vi "LoadInstrFunc.vi"(8 "ErrorIn(No Error)":errorcluster caption="entrée d'erreur (pas d'erreur)", 9 "New Instr":bool, 10 "LoadInstr":T1, 11 "Experiment.lvclass":refnum<class "Experiment.lvclass">) -> (0 "sortie d'erreur":errorcluster, 3 "Experiment.lvclass Out":refnum<class "Experiment.lvclass">)   [LabVIEW 2019, in "Experiment.lvclass"]
uses:
  Experiment.lvclass
  LoadInstr.ctl
  Experiment.lvclass/Experiment.ctl
  DevicesClass/BaseDevice/BaseDevice.lvclass
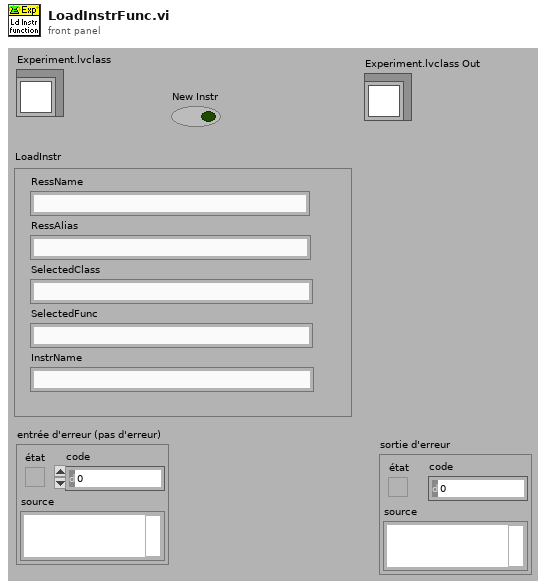
[diagram p1: front panel]
types:
  T1 = typedef "LoadInstr.ctl" = cluster{"SelectedClass":string, "SelectedFunc":string, "InstrName":string, "RessAlias":string, "RessName":string}
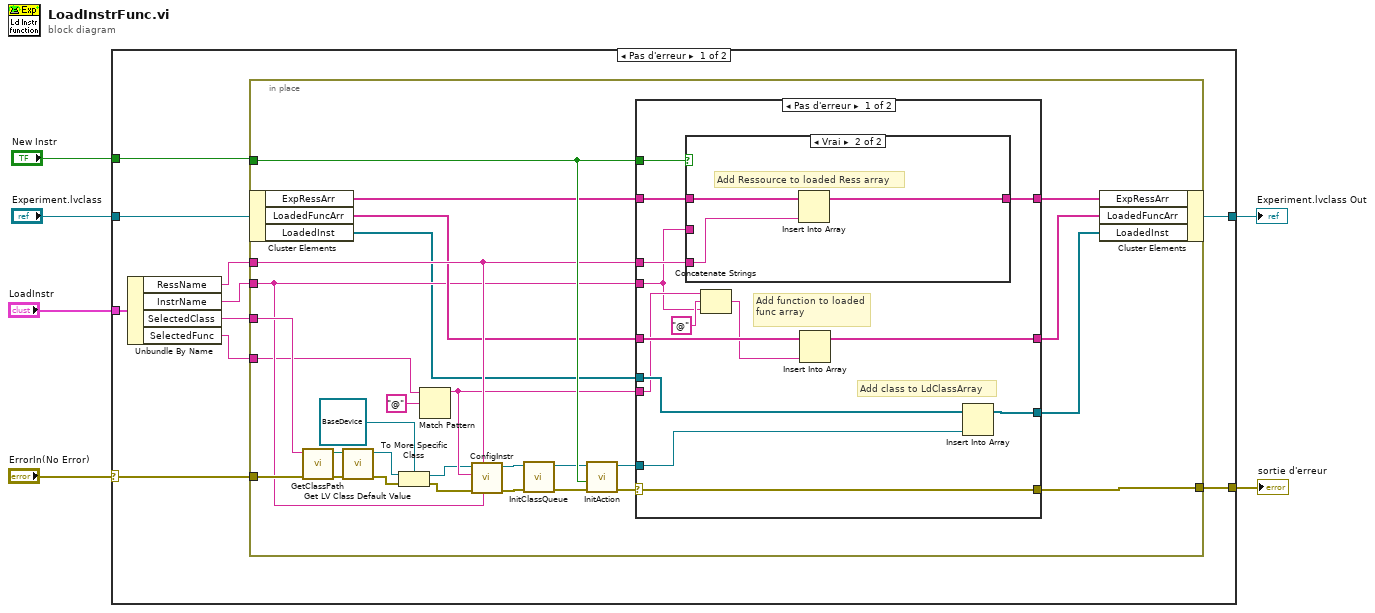
[diagram p0: block diagram]
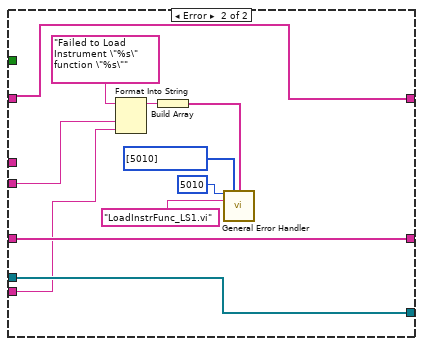
[diagram p3: hidden frame]
diagram:
  n1 = case shown="Pas d'erreur" "ErrorIn(No Error)" {
    selector: "ErrorIn(No Error)" -> [w16 w75]
    tunnel: [w15 w75] -> w5
    tunnel: "New Instr" -> [w14 _]
    tunnel: "Experiment.lvclass" -> [w12 w74]
    tunnel: [w13 w74] -> w2
    tunnel: "LoadInstr" -> [w7 _]
    frame No Error {
      n2 = Unbundle By Name(w7) -> ("RessName"=w11:string, "InstrName"=w10:string, "SelectedClass"=w9:string, "SelectedFunc"=w8:string)
      n3 = in-place {
        in-place-border: w16 -> [w40]
        in-place-border: w9 -> [w39]
        in-place-border: w11 -> [w33]
        in-place-border: w8 -> [w26]
        in-place-border: w10 -> [w28]
        in-place-border: [w38] -> w15
        in-place-border: w14 -> [w37]
        n4 = in-place-cluster #1(w12) -> ("ExpRessArr"=w34:string[], "LoadedFuncArr"=w30:string[], "LoadedInst"=w17:refnum<class "BaseDevice.lvclass">[])
        n5 = call "GetClassPath.vi"("error in (no error)"=w40, "ClassName"=w39) -> ("error out"=w41:errorcluster, "ClassPath"=w42:path)  [unwired: 7 in, 1 out]
        n6 = call <vilib>:"Get LV Class Default Value.vi"("error in (no error)"=w41, "class path"=w42) -> ("error out"=w23:errorcluster, "object"=w44:refnum<class>)  [unwired: 8 in]
        n7 = To More Specific Class(target class=refnum<class "BaseDevice.lvclass"> refnum ("Device.lvclass"), reference=w44, error in=w23) -> (specific class reference=w24:refnum<class "BaseDevice.lvclass">, error out=w22:errorcluster)
        n8 = Match Pattern(string=w26, regular expression="@" ("chaîne")) -> (before substring=w25:string)  [unwired: 1 in, 3 out]
        n9 = call-dynamic "ConfigInstr.vi"("InstrumentName"=w28, "VisaRessIn"=w33, "error in (no error)"=w22, "Function"=w25, "Device en entrée"=w24) -> ("error out"=w21:errorcluster, "Device en sortie"=w19:refnum<class "BaseDevice.lvclass">)  [unwired: 5 in]
        n10 = call "InitClassQueue.vi"("ErrorIn(No Error)"=w21, "BaseDevice.lvclass"=w19) -> ("sortie d'erreur"=w20:errorcluster, "BaseDevice.lvclass Out"=w18:refnum<class "BaseDevice.lvclass">)  [unwired: 6 in, 2 out]
        n11 = call-dynamic "InitAction.vi"("error in (no error)"=w20, "FirstClassInst"=w37, "Device en entrée"=w18) -> ("error out"=w35:errorcluster, "Device en sortie"=w36:refnum<class "BaseDevice.lvclass">)  [unwired: 7 in]
        n12 = case shown="Pas d'erreur" w35 {
          selector: w35 -> [w53 _]
          tunnel: [w46 w66] -> w29
          tunnel: [w58 w73] -> w31
          tunnel: w30 -> [w57 w73]
          tunnel: w33 -> [w56 _]
          tunnel: w34 -> [w55 w64]
          tunnel: w36 -> [w45 _]
          tunnel: w37 -> [w54 _]
          tunnel: [w53 _] -> w38
          tunnel: [w52 w64] -> w32
          tunnel: w17 -> [w51 w66]
          tunnel: w28 -> [w47 w65]
          tunnel: w25 -> [w50 w63]
          frame No Error {
            # "Add class to LdClassArray"
            # "Add function to loaded func array"
            n13 = case shown="Vrai" w54 {
              tunnel: w56 -> [_ w62]
              tunnel: [w59 w61] -> w52
              tunnel: w55 -> [w59 w60]
              tunnel: w47 -> [_ _]
              frame False {
              }
              frame True {
                # "Add Ressource to loaded Ress array"
                n14 = Insert Into Array(array=w60, new element=w62) -> (w61:string[])  [unwired: 1 in]
              }
            }
            n15 = Concatenate Strings(w50, "@" ("chaîne"), w47) -> (w48:string)
            n16 = Insert Into Array(array=w57, new element=w48) -> (w58:string[])  [unwired: 1 in]
            n17 = Insert Into Array(array=w51, new element=w45) -> (w46:refnum<class "BaseDevice.lvclass">[])  [unwired: 1 in]
          }
          frame Error {
            n18 = Format Into String(format string="Failed to Load Instrument \"%s\" function \"%s\"" ("[error source] (\" \")"), w65, w63) -> (resulting string=w70:string)  [unwired: 2 in, 1 out]
            n19 = Build Array(w70) -> (w71:string[])
            n20 = call <vilib>:"General Error Handler.vi"("[error code] (0)"=5010, "[user-defined codes]"=i32[] [5010], "[user-defined descriptions]"=w71, "[error source] (\" \")"="LoadInstrFunc_LS1.vi" ("[error source] (\" \")")) -> ()  [unwired: 7 in, 5 out]
          }
        }
        n21 = in-place-cluster #1("ExpRessArr"=w32, "LoadedFuncArr"=w31, "LoadedInst"=w29) -> (w13:refnum<class "Experiment.lvclass">)
      }
    }
    frame Error {
      # "operation canceled"
    }
  }
  "sortie d'erreur" <- w5
  "Experiment.lvclass Out" <- w2
